vi "CCM-Enumerate Endpoints.vi"(0 "Path In":path, 11 "error in (no error)":errorcluster) -> (4 "Path Out":path, 6 "Analog":cluster{"Out":string[], "In":string[]}, 10 "Digital":cluster{"Out":string[], "In":string[]}, 14 "Endpoints":cluster{"Name":string[]}[](array[cluster]), 15 "error out":errorcluster)   [LabVIEW 2020]
uses:
  <vilib>/Utility/config.llb/NI_LVConfig.lvlib
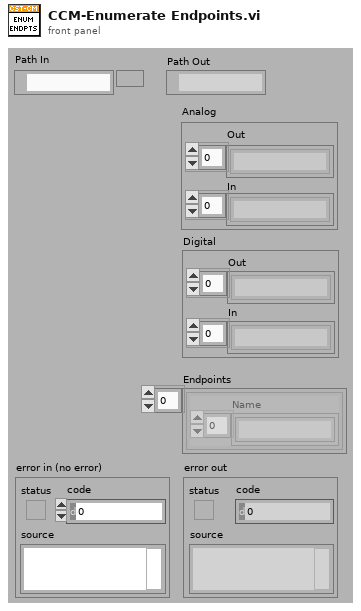
[diagram p1: front panel]
types:
  T1 = typedef "NI_LVConfig.lvlib/Config Data RefNum.ctl" = refnum<k1>
  T2 = cluster{"key names":string[], "key names":string[]}
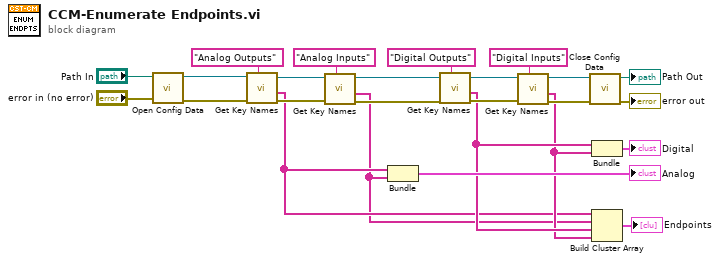
[diagram p0: block diagram]
diagram:
  n1 = call <vilib>:"Open Config Data.vi"("error in (no error)"="error in (no error)", "configuration file path"="Path In") -> ("error out"=w21:errorcluster, "refnum"=w22:T1)  [unwired: 7 in, 1 out]
  n2 = call <vilib>:"Get Key Names.vi"("section"="Analog Outputs", "error in (no error)"=w21, "refnum"=w22) -> ("error out"=w19:errorcluster, "key names"=w2:string[], "refnum out"=w18:T1)  [unwired: 5 in, 1 out]
  n3 = call <vilib>:"Get Key Names.vi"("section"="Analog Inputs", "error in (no error)"=w19, "refnum"=w18) -> ("error out"=w11:errorcluster, "key names"=w1:string[], "refnum out"=w12:T1)  [unwired: 5 in, 1 out]
  n4 = Bundle("key names"=w2, "key names"=w1) -> (→"Analog":T2)  [unwired: 1 in]
  n5 = call <vilib>:"Get Key Names.vi"("section"="Digital Outputs", "error in (no error)"=w11, "refnum"=w12) -> ("error out"=w10:errorcluster, "key names"=w4:string[], "refnum out"=w14:T1)  [unwired: 5 in, 1 out]
  n6 = call <vilib>:"Get Key Names.vi"("section"="Digital Inputs", "error in (no error)"=w10, "refnum"=w14) -> ("error out"=w7:errorcluster, "key names"=w3:string[], "refnum out"=w8:T1)  [unwired: 5 in, 1 out]
  n7 = call <vilib>:"Close Config Data.vi"("error in (no error)"=w7, "refnum"=w8) -> ("error out"=→"error out":errorcluster, "file path"=→"Path Out":path)  [unwired: 8 in]
  n8 = Bundle("key names"=w4, "key names"=w3) -> (→"Digital":T2)  [unwired: 1 in]
  n9 = Build Cluster Array(w2, w1, w4, w3) -> (→"Endpoints":cluster{"key names":string[]}[])
